vi "Start Sequence Acquisition.vi"(8 "error in (no error)":errorcluster, 11 "Stage in":refnum<class "Stage.lvclass">) -> (0 "error out":errorcluster, 3 "Stage out":refnum<class "Stage.lvclass">)   [LabVIEW 2020, in "Stage.lvlib" / "Stage.lvclass"]
uses:
  Stage.lvclass
  C:/Program Files/National Instruments/LabVIEW 2020/vi.lib/ActorFramework/Actor/Actor.lvclass
  Stage.lvclass/Stage.ctl
  <vilib>/ActorFramework/Actor/Actor.lvclass/Actor.ctl
  <vilib>/ActorFramework/Message Enqueuer/Message Enqueuer.lvclass/Message Enqueuer.ctl
  <vilib>/ActorFramework/Message Enqueuer/Init from Existing Queue.vi
  <vilib>/ActorFramework/Message Enqueuer/Enqueue.vi
  Stage Messages/Start Sequence Acquisition Msg/Start Sequence Acquisition Msg.lvclass
  C:/Program Files/National Instruments/LabVIEW 2020/vi.lib/ActorFramework/Message/Message.lvclass
  <vilib>/ActorFramework/Message Priority Queue/Priority Enqueue.vi
  <vilib>/ActorFramework/Message Enqueuer/Message Enqueuer.lvclass
  <vilib>/ActorFramework/Actor/Actor.lvclass
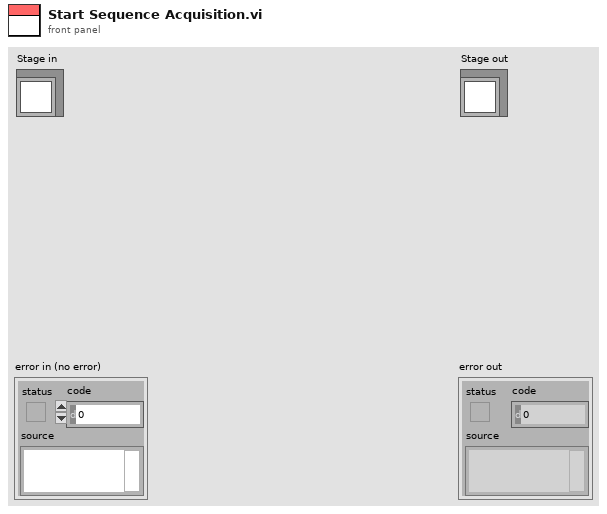
[diagram p1: front panel]
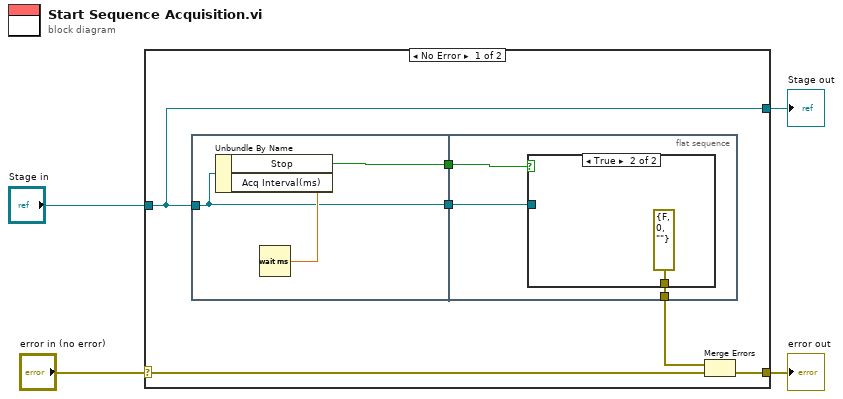
[diagram p0: block diagram]
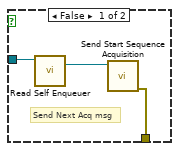
[diagram p2: hidden frame]
diagram:
  n1 = case shown="No Error" "error in (no error)" {
    selector: "error in (no error)" -> [w9 w22]
    tunnel: [w10 w22] -> w3
    tunnel: [w6 w21] -> w1
    tunnel: "Stage in" -> [w6 w21]
    frame No Error {
      n2 = flat-sequence {
        tunnel: w6 -> [w11]
        tunnel: [w13] -> w8
        tunnel: [w11] -> w7
        tunnel: w8 -> [w16]
        tunnel: w7 -> [w15]
        tunnel: [w14] -> w5
        frame #0 {
          n3 = Unbundle By Name(w11) -> ("Stop"=w13:bool, "Acq Interval(ms)"=w12:dbl)
          n4 = Wait (ms)(milliseconds to wait=w12) -> ()  [unwired: 1 out]
        }
        frame #1 {
          n5 = case shown="True" w16 {
            tunnel: w15 -> [w18 _]
            tunnel: [w17 errorcluster {"status"=FALSE, "code"=0, "source"=""} ("error out")] -> w14
            frame False {
              # "Send Next Acq msg"
              n6 = call <vilib>:"Read Self Enqueuer.vi"("Actor"=w18) -> ("Self Enqueuer"=w19:refnum<class "Message Enqueuer.lvclass">)  [unwired: 10 in]
              n7 = call "Send Start Sequence Acquisition.vi"("Message Enqueuer"=w19) -> ("error out"=w17:errorcluster)  [unwired: 9 in, 1 out]
            }
            frame True {
            }
          }
        }
      }
      n8 = Merge Errors(w5, w9) -> (w10:errorcluster)
    }
    frame Error {
    }
  }
  "error out" <- w3
  "Stage out" <- w1
